vi "write_panel_number.vi"(8 "error in (no error)":errorcluster, 10 "panel_number":T1, 11 "panel in":refnum<class "panel.lvclass">) -> (0 "error out":errorcluster, 3 "panel out":refnum<class "panel.lvclass">)   [LabVIEW 2015, in "panel.lvclass"]
uses:
  panel.lvclass
  front_panel_class/hardware_caller_queue_numbers.ctl
  panel.lvclass/panel.ctl
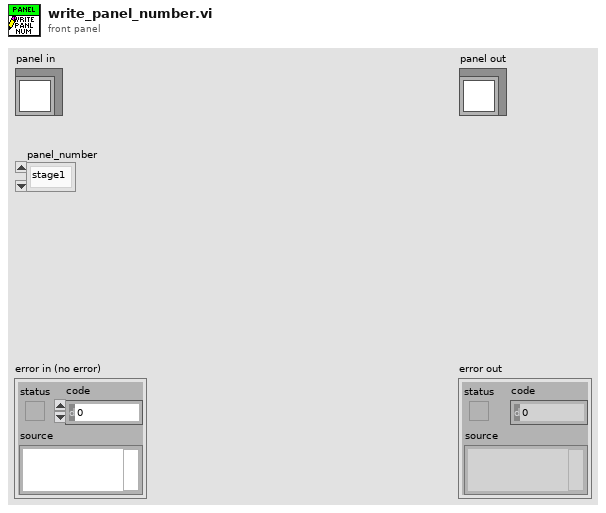
[diagram p1: front panel]
types:
  T1 = typedef "hardware_caller_queue_numbers.ctl" = enum16{"stage1", "stage2", "experiment", "detector"}
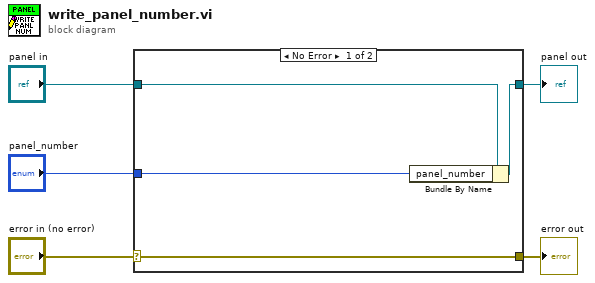
[diagram p0: block diagram]
diagram:
  n1 = case shown="No Error" "error in (no error)" {
    selector: "error in (no error)" -> [w9 w10]
    tunnel: [w9 w10] -> w4
    tunnel: [w7 w11] -> w2
    tunnel: "panel in" -> [w8 w11]
    tunnel: "panel_number" -> [w6 _]
    frame No Error {
      n2 = Bundle By Name(cluster=w8, "panel_number"=w6) -> (w7:refnum<class "panel.lvclass">)
    }
    frame Error {
    }
  }
  "error out" <- w4
  "panel out" <- w2
